vi "OpenFile.vi"(8 "error in (no error)":errorcluster, 10 "File Path":path) -> (0 "error out":errorcluster, 3 "RWFile out":refnum<class "RWFile.lvclass">)   [LabVIEW 2021, in "RWFile.lvclass"]
uses:
  RWFile.lvclass
  RWFile.lvclass/RWFile.ctl
  File/File.lvclass
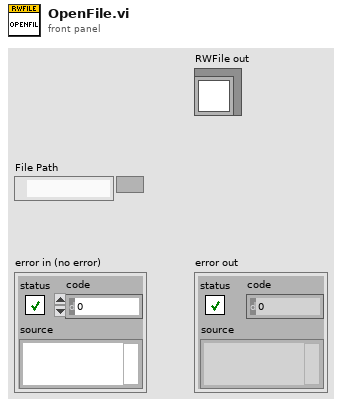
[diagram p1: front panel]
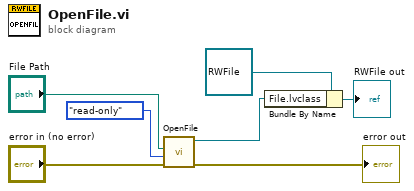
[diagram p0: block diagram]
diagram:
  n1 = call "OpenFile.vi"("error in (no error)"="error in (no error)", "access (0:read/write)"=enum16{"read/write", "read-only", "write-only"}."read-only", "File Path"="File Path") -> ("error out"=→"error out":errorcluster, "File out"=w1:refnum<class "File.lvclass">)  [unwired: 7 in]
  n2 = Bundle By Name(cluster=refnum<class "RWFile.lvclass"> refnum ("ROFile in"), "File.lvclass"=w1) -> (→"RWFile out":refnum<class "RWFile.lvclass">)
